vi "Change in Custom Actions.vi"(8 "error in (no error)":errorcluster, 10 "Custom Actions":cluster{"Key":string, "Timing":string}[](array[cluster]), 11 "Bundle Builder in":refnum<class "Bundle Builder.lvclass">) -> (0 "error out":errorcluster, 1 "Custom Actions File Names":string[](array[string]), 2 "Product List File Names":string[](array[string]), 3 "Bundle Builder out":refnum<class "Bundle Builder.lvclass">, 4 "Bundle Filename":string)   [LabVIEW 2020, in "Bundle Builder.lvclass"]
uses:
  Bundle Builder.lvclass
  Bundle Builder.lvclass/Bundle Builder.ctl
  4f63f28f-5265-4602-8317-7e5f909f2807.vi
  5d65ce95-3f27-4ad9-b4d3-753b2ea8e44f.vi
  <vilib>/Comparison/Equal/Equal Functor/Equal Functor.lvclass
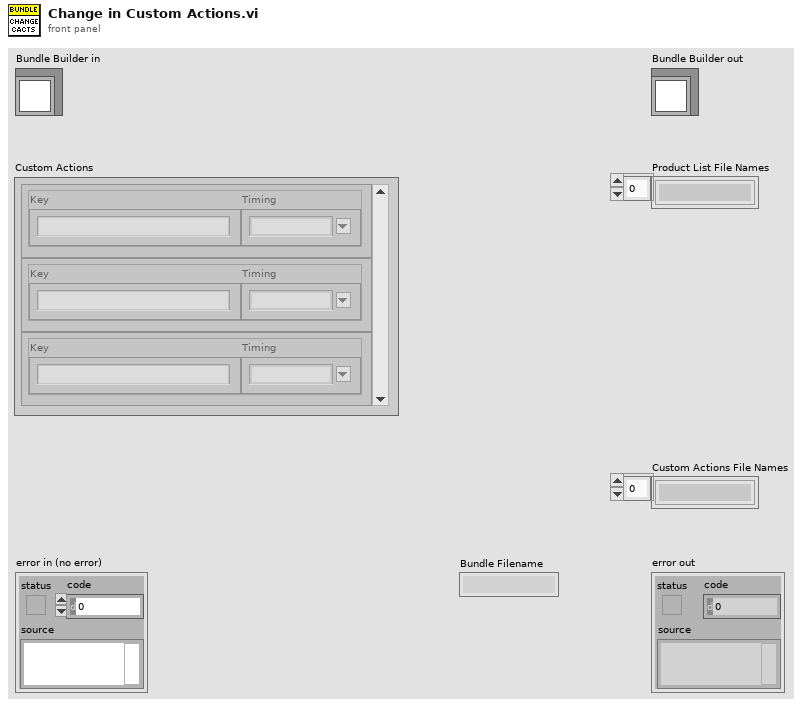
[diagram p1: front panel]
types:
  T1 = enum16{"All Elements Deleted", "Element Deleted", "Element Inserted", "Element Content Changed"}
  T2 = cluster{"Display Name":string, "Commands":cluster{"Path":string, "Parameters":string, "Successful Exit Codes":string, "Log Command":cluster{"Flag":string, "File Name":string}}[]}[]
  T3 = cluster{"Display Name":string, "Commands":cluster{"Path":string, "Parameters":string, "Successful Exit Codes":string, "Log Command":cluster{"Flag":string, "File Name":string}}[]}
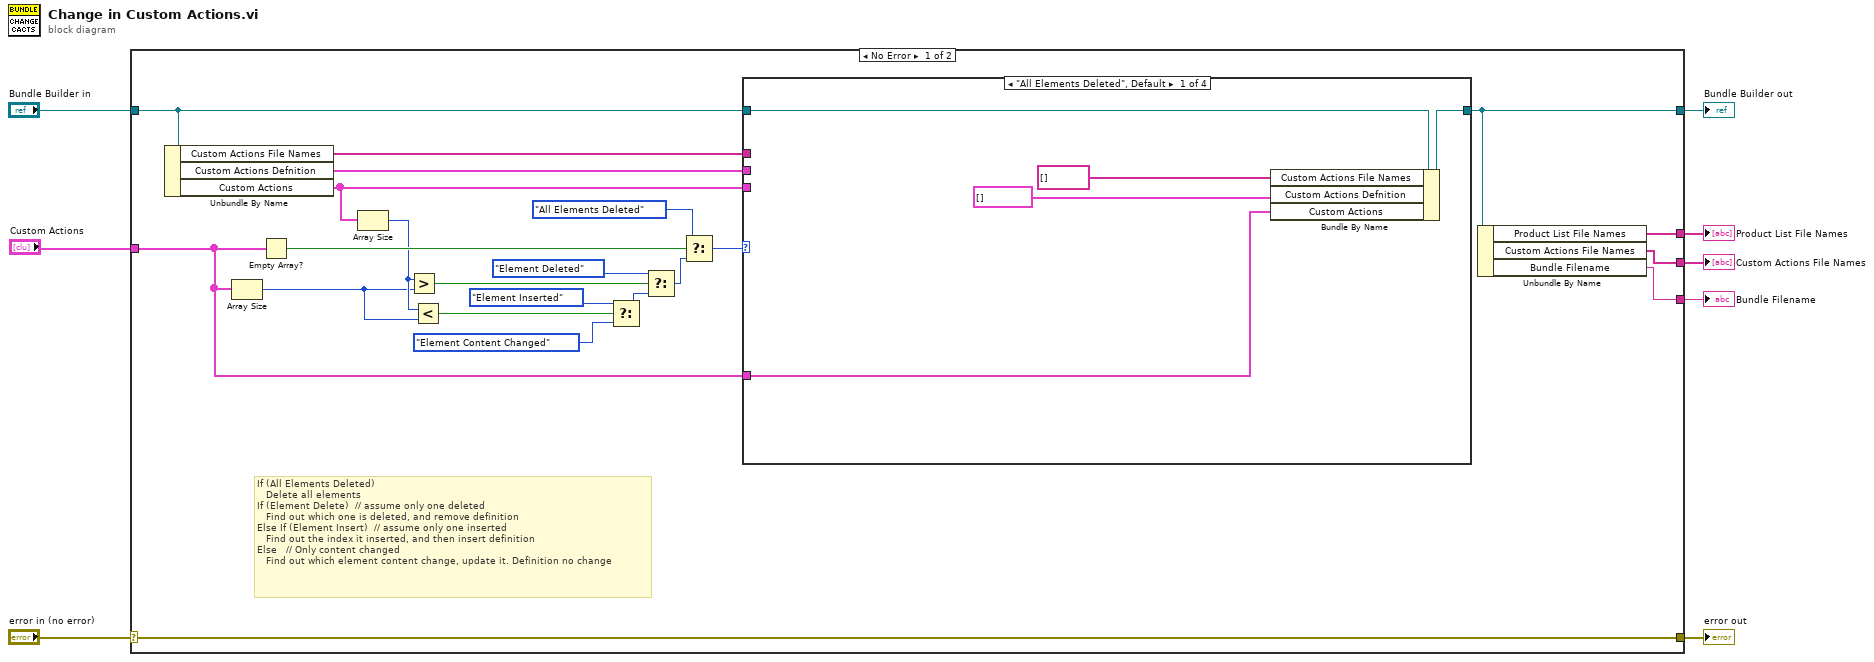
[diagram p0: block diagram]
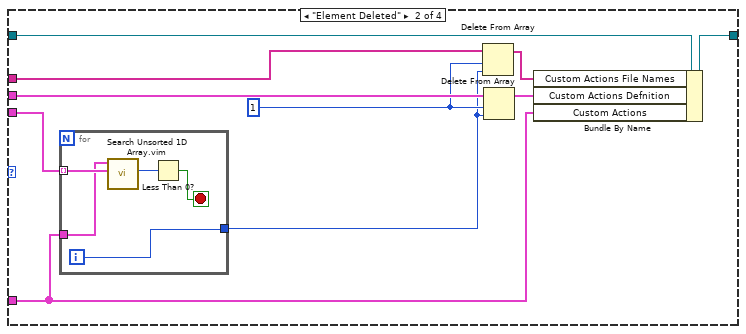
[diagram p2: hidden frame]
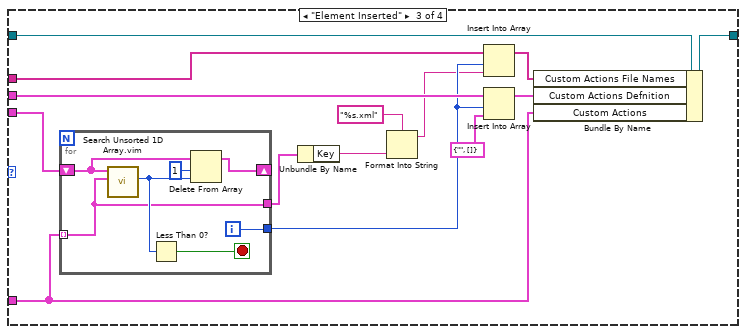
[diagram p3: hidden frame]
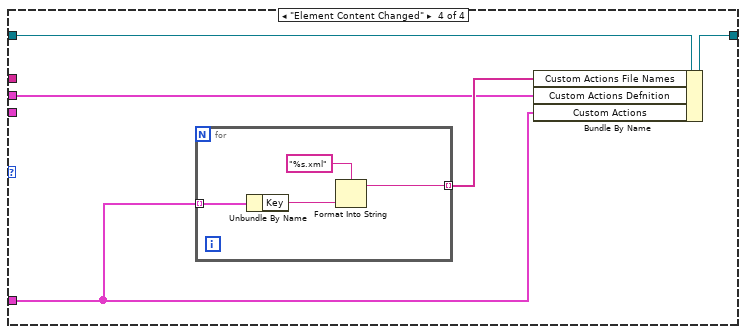
[diagram p4: hidden frame]
diagram:
  n1 = case shown="No Error" "error in (no error)" {
    selector: "error in (no error)" -> [w30 w82]
    tunnel: [w30 w82] -> w7
    tunnel: [w13 w81] -> w5
    tunnel: "Bundle Builder in" -> [w17 w81]
    tunnel: "Custom Actions" -> [w16 _]
    tunnel: [w11 _] -> w4
    tunnel: [w10 _] -> w3
    tunnel: [w9 _] -> w2
    frame No Error {
      # "If (All Elements Deleted)\n   Delete all elements\nIf (Element Delete)  // assume only one deleted\n   Find out which one is deleted, and remove definition\nElse If (Element Insert)  // assume only one inserted\n   Find out the index it inserted, and then insert definition\nElse   // Only content changed\n   Find out which element content change, update it. Definition no change"
      n2 = Unbundle By Name(w17) -> ("Custom Actions File Names"=w12:string[], "Custom Actions Defnition"=w14:T2, "Custom Actions"=w15:cluster{"Key":string, "Timing":string}[])
      n3 = Array Size(array=w16) -> (size(s)=w23:i32)
      n4 = Empty Array?(array=w16) -> (empty?=w29:bool)
      n5 = Array Size(array=w15) -> (size(s)=w24:i32)
      n6 = Greater?(x=w24, y=w23) -> (0:w25:bool)
      n7 = Less?(x=w24, y=w23) -> (x < y?=w20:bool)
      n8 = Select(t=T1."Element Inserted", s=w20, f=T1."Element Content Changed") -> (s? t:f=w22:T1)
      n9 = Select(t=T1."Element Deleted", s=w25, f=w22) -> (s? t:f=w26:T1)
      n10 = Select(t=T1."All Elements Deleted", s=w29, f=w26) -> (s? t:f=w18:T1)
      n11 = case shown="\"All Elements Deleted\", Default" w18 {
        tunnel: w17 -> [w35 w45 w64 w76]
        tunnel: [w34 w44 w63 w75] -> w13
        tunnel: w16 -> [w33 w41 w60 w74]
        tunnel: w15 -> [_ w43 w62 _]
        tunnel: w14 -> [_ w42 w61 w72]
        tunnel: w12 -> [_ w40 w59 _]
        frame "All Elements Deleted", Default {
          n12 = Bundle By Name(cluster=w35, "Custom Actions File Names"=string[] [] ("Product List File Names"), "Custom Actions Defnition"=T2 [], "Custom Actions"=w33) -> (w34:refnum<class "Bundle Builder.lvclass">)
        }
        frame "Element Deleted" {
          w38 = 1 ("length")
          n13 = for {
            tunnel: w43 -> [w50] mode=indexing
            tunnel: w41 -> [w49]
            tunnel: [w46] -> w37
            i -> [w46]
            stop <- w48 stop-if-true
            n14 = call "Search Unsorted 1D Array.vim"("element"=w50, "unsorted 1D array"=w49) -> ("index of element"=w47:i32)  [unwired: 9 in]
            n15 = Less Than 0?(x=w47) -> (x < 0?=w48:bool)
          }
          n16 = Delete From Array(array=w40, length=w38, index=w37) -> (array with subset deleted=w39:string[])  [unwired: 1 out]
          n17 = Delete From Array(array=w42, length=w38, index=w37) -> (array with subset deleted=w36:T2)  [unwired: 1 out]
          n18 = Bundle By Name(cluster=w45, "Custom Actions File Names"=w39, "Custom Actions Defnition"=w36, "Custom Actions"=w41) -> (w44:refnum<class "Bundle Builder.lvclass">)
        }
        frame "Element Inserted" {
          n19 = for {
            tunnel: w60 -> [w65] mode=indexing
            tunnel: [w70] -> w58
            shift-right: [w66] -> _
            shift-left: w62 -> [w69]
            tunnel: [w65] -> w57
            i -> [w70]
            stop <- w71 stop-if-true
            n20 = call "Search Unsorted 1D Array.vim"("element"=w65, "unsorted 1D array"=w69) -> ("index of element"=w68:i32)  [unwired: 9 in]
            n21 = Less Than 0?(x=w68) -> (x < 0?=w71:bool)
            n22 = Delete From Array(array=w69, length=1, index=w68) -> (array with subset deleted=w66:cluster{"Key":string, "Timing":string}[])  [unwired: 1 out]
          }
          n23 = Unbundle By Name(w57) -> ("Key"=w55:string)
          n24 = Format Into String(format string="%s.xml", w55) -> (resulting string=w54:string)  [unwired: 2 in, 1 out]
          n25 = Insert Into Array(array=w59, index=w58, new element=w54) -> (w53:string[])
          n26 = Insert Into Array(array=w61, index=w58, new element=T3 {"Display Name"="", "Commands"=[]} ("Custom Actions")) -> (w52:T2)
          n27 = Bundle By Name(cluster=w64, "Custom Actions File Names"=w53, "Custom Actions Defnition"=w52, "Custom Actions"=w60) -> (w63:refnum<class "Bundle Builder.lvclass">)
        }
        frame "Element Content Changed" {
          n28 = for {
            tunnel: w74 -> [w78] mode=indexing
            tunnel: [w77] -> w73 mode=indexing
            n29 = Unbundle By Name(w78) -> ("Key"=w79:string)
            n30 = Format Into String(format string="%s.xml", w79) -> (resulting string=w77:string)  [unwired: 2 in, 1 out]
          }
          n31 = Bundle By Name(cluster=w76, "Custom Actions File Names"=w73, "Custom Actions Defnition"=w72, "Custom Actions"=w74) -> (w75:refnum<class "Bundle Builder.lvclass">)
        }
      }
      n32 = Unbundle By Name(w13) -> ("Product List File Names"=w11:string[], "Custom Actions File Names"=w10:string[], "Bundle Filename"=w9:string)
    }
    frame Error {
    }
  }
  "error out" <- w7
  "Bundle Builder out" <- w5
  "Product List File Names" <- w4
  "Custom Actions File Names" <- w3
  "Bundle Filename" <- w2
